vi "PC Hard.vi"(11 "DataIn":T1) -> (3 "DataOut":T1)   [LabVIEW 2017]
doc: "SubVI criada para realizar o movimento do BOT em caso de partida Player 1 x PC no nível difícil"
uses:
  controls/TabuleiroCoordenadas.ctl
  controls/GameOption.ctl
  controls/Tabuleiro.ctl
  controls/DataIn.ctl
  controls/Table.ctl
  MatchDataClasses/MatchData/MatchData.lvclass
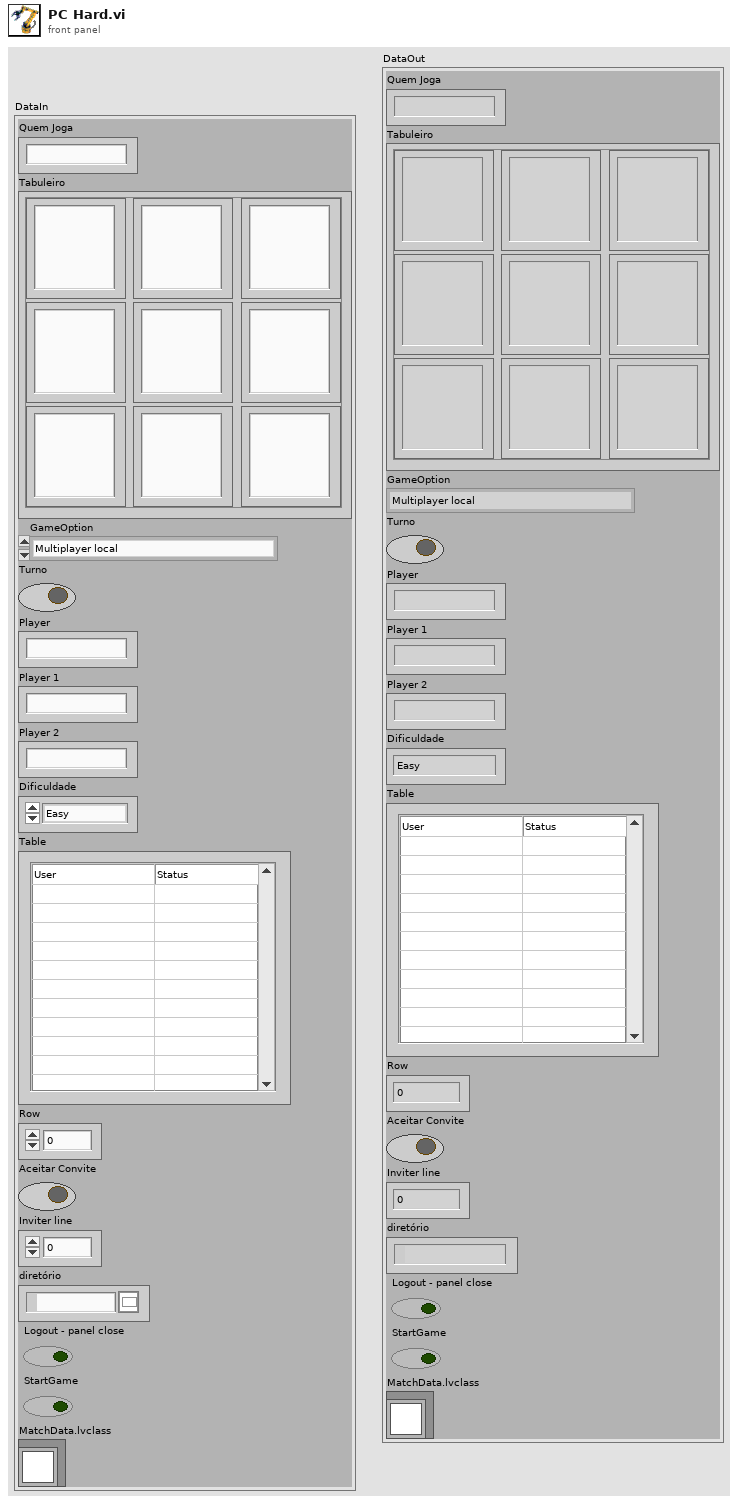
[diagram p1: front panel]
types:
  T1 = typedef "DataIn.ctl" = cluster{"Quem Joga":string, "Tabuleiro":T2, "GameOption":T3, "Turno":bool, "Player":string, "Player 1":string, "Player 2":string, "Dificuldade":enum16{"Easy", "Medium", "Hard"}, "Table":T4, "Row":u32, "Aceitar Convite":bool, "Inviter line":u32, "diretório":path, "Logout - panel close":bool, "StartGame":bool, "MatchData.lvclass":refnum<class "MatchData.lvclass">}
  T2 = typedef "Tabuleiro.ctl" = cluster{"(0,0)":string, "(1,0)":string, "(0,1)":string, "(1,1)":string, "(2,0)":string, "(1,2)":string, "(2,2)":string, "(0,2)":string, "(2,1) ":string}
  T3 = typedef "GameOption.ctl" = enum16{"Multiplayer local", "Multiplayer remoto", "Single Player", "Wait for Event", "Initialize", "Stop"}
  T4 = typedef "Table.ctl" = string[][]
  T5 = typedef "TabuleiroCoordenadas.ctl" = enum16{"0,0", "0,1", "0,2", "1,0", "1,1", "1,2", "2,0", "2,1", "2,2"}
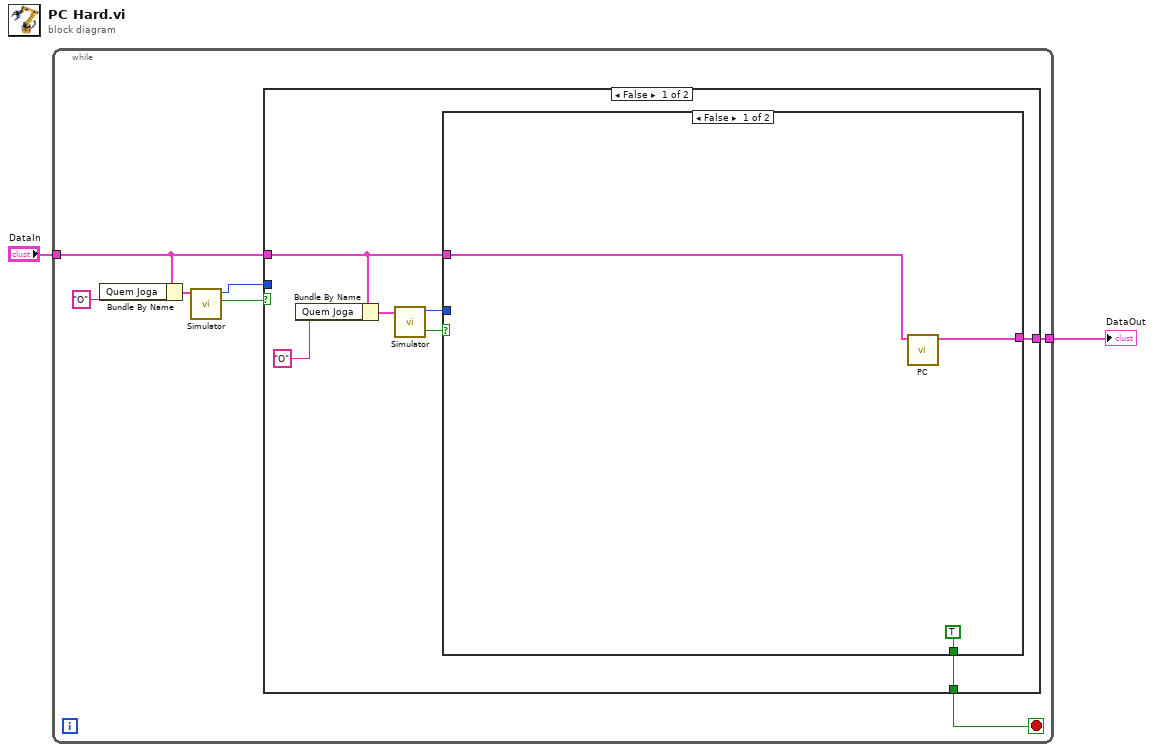
[diagram p0: block diagram]
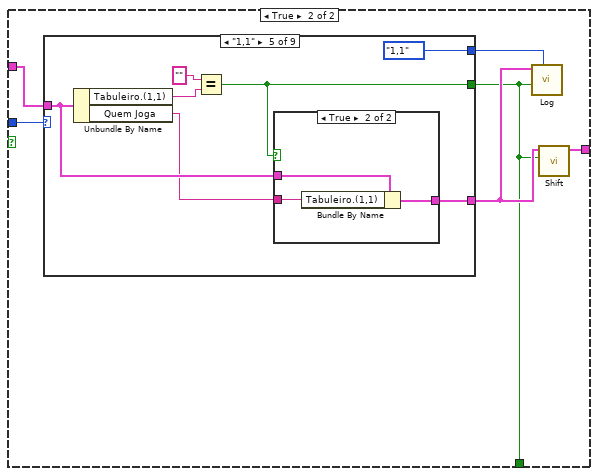
[diagram p2: hidden frame]
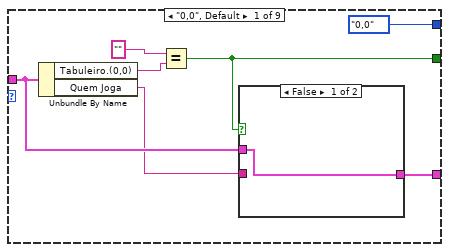
[diagram p3: hidden frame]
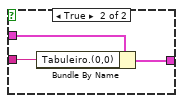
[diagram p4: hidden frame]
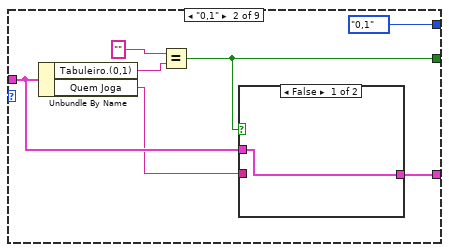
[diagram p5: hidden frame]
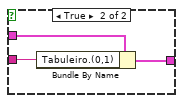
[diagram p6: hidden frame]
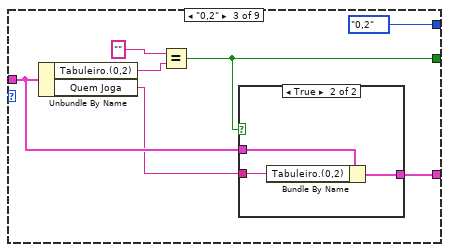
[diagram p7: hidden frame]
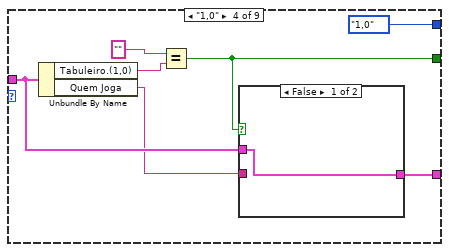
[diagram p9: hidden frame]
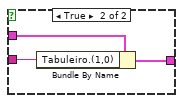
[diagram p10: hidden frame]
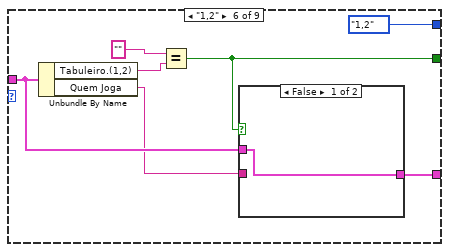
[diagram p12: hidden frame]
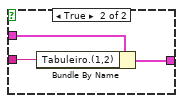
[diagram p13: hidden frame]
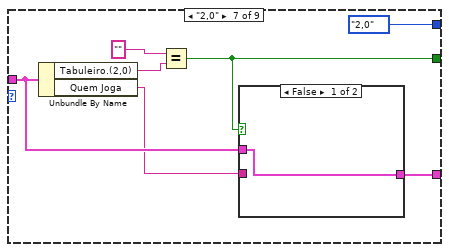
[diagram p14: hidden frame]
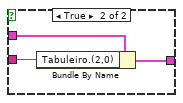
[diagram p15: hidden frame]
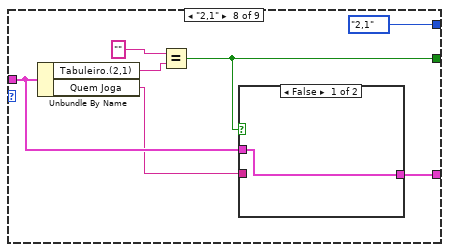
[diagram p16: hidden frame]
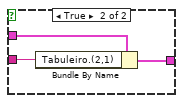
[diagram p17: hidden frame]
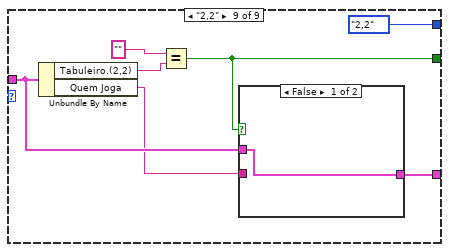
[diagram p18: hidden frame]
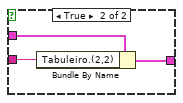
[diagram p19: hidden frame]
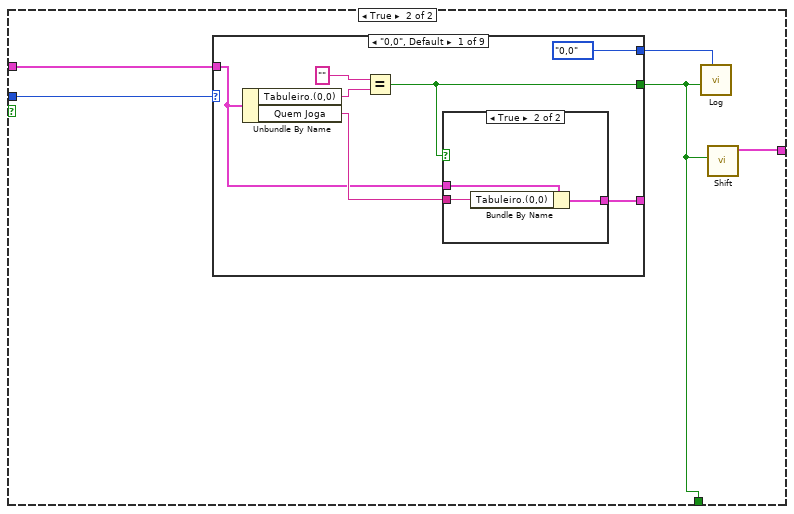
[diagram p20: hidden frame]
diagram:
  n1 = while {
    tunnel: [w9] -> w1
    tunnel: "DataIn" -> [w5]
    stop <- w4 stop-if-true
    n2 = Bundle By Name(cluster=w5, "Quem Joga"="O") -> (w6:T1)
    n3 = call "Simulator.vi"("DataIn"=w6) -> ("true = ganhou"=w8:bool, "Enum"=w3:T5)  [unwired: 9 in]
    n4 = case shown="False" w8 {
      tunnel: [w16 w129] -> w9
      tunnel: w5 -> [w11 w126]
      tunnel: [w13 w125] -> w4
      tunnel: w3 -> [_ w127]
      frame False {
        n5 = Bundle By Name(cluster=w11, "Quem Joga"="O") -> (w12:T1)
        n6 = call "Simulator.vi"("DataIn"=w12) -> ("true = ganhou"=w14:bool, "Enum"=w15:T5)  [unwired: 9 in]
        n7 = case shown="False" w14 {
          tunnel: w15 -> [_ w25]
          tunnel: w11 -> [w18 w24]
          tunnel: [w19 w21] -> w16
          tunnel: [TRUE w20] -> w13
          frame False {
            n8 = call "PC.vi"("DataIn"=w18) -> ("DataOut"=w19:T1)  [unwired: 10 in]
          }
          frame True {
            n9 = case shown="\"1,1\"" w25 {
              tunnel: w24 -> [w29 w40 w51 w62 w73 w84 w95 w106 w117]
              tunnel: [w30 w41 w52 w63 w74 w85 w96 w107 w118] -> w20
              tunnel: [w27 w38 w49 w60 w71 w82 w93 w104 w115] -> w22
              tunnel: [TabuleiroCoordenadas."0,0" ("Enum") TabuleiroCoordenadas."0,1" ("Enum") TabuleiroCoordenadas."0,2" ("Enum") TabuleiroCoordenadas."1,0" ("Enum") TabuleiroCoordenadas."1,1" ("Enum") TabuleiroCoordenadas."1,2" ("Enum") TabuleiroCoordenadas."2,0" ("Enum") TabuleiroCoordenadas."2,1" ("Enum") TabuleiroCoordenadas."2,2" ("Enum")] -> w23
              frame "0,0", Default {
                n10 = Unbundle By Name(w29) -> ("Tabuleiro.(0,0)"=w32:string, "Quem Joga"=w28:string)
                n11 = Equal?(x="", y=w32) -> (x = y?=w30:bool)
                n12 = case shown="False" w30 {
                  tunnel: w29 -> [w33 w36]
                  tunnel: w28 -> [_ w35]
                  tunnel: [w33 w34] -> w27
                  frame False {
                  }
                  frame True {
                    n13 = Bundle By Name(cluster=w36, "Tabuleiro.(0,0)"=w35) -> (w34:T1)
                  }
                }
              }
              frame "0,1" {
                n14 = Unbundle By Name(w40) -> ("Tabuleiro.(0,1)"=w43:string, "Quem Joga"=w39:string)
                n15 = Equal?(x="", y=w43) -> (x = y?=w41:bool)
                n16 = case shown="False" w41 {
                  tunnel: w40 -> [w44 w47]
                  tunnel: w39 -> [_ w46]
                  tunnel: [w44 w45] -> w38
                  frame False {
                  }
                  frame True {
                    n17 = Bundle By Name(cluster=w47, "Tabuleiro.(0,1)"=w46) -> (w45:T1)
                  }
                }
              }
              frame "0,2" {
                n18 = Unbundle By Name(w51) -> ("Tabuleiro.(0,2)"=w54:string, "Quem Joga"=w50:string)
                n19 = Equal?(x="", y=w54) -> (x = y?=w52:bool)
                n20 = case shown="True" w52 {
                  tunnel: w51 -> [w55 w58]
                  tunnel: w50 -> [_ w57]
                  tunnel: [w55 w56] -> w49
                  frame False {
                  }
                  frame True {
                    n21 = Bundle By Name(cluster=w58, "Tabuleiro.(0,2)"=w57) -> (w56:T1)
                  }
                }
              }
              frame "1,0" {
                n22 = Unbundle By Name(w62) -> ("Tabuleiro.(1,0)"=w65:string, "Quem Joga"=w61:string)
                n23 = Equal?(x="", y=w65) -> (x = y?=w63:bool)
                n24 = case shown="False" w63 {
                  tunnel: w62 -> [w66 w69]
                  tunnel: w61 -> [_ w68]
                  tunnel: [w66 w67] -> w60
                  frame False {
                  }
                  frame True {
                    n25 = Bundle By Name(cluster=w69, "Tabuleiro.(1,0)"=w68) -> (w67:T1)
                  }
                }
              }
              frame "1,1" {
                n26 = Unbundle By Name(w73) -> ("Tabuleiro.(1,1)"=w76:string, "Quem Joga"=w72:string)
                n27 = Equal?(x="", y=w76) -> (x = y?=w74:bool)
                n28 = case shown="True" w74 {
                  tunnel: w73 -> [w77 w80]
                  tunnel: w72 -> [_ w79]
                  tunnel: [w77 w78] -> w71
                  frame False {
                  }
                  frame True {
                    n29 = Bundle By Name(cluster=w80, "Tabuleiro.(1,1)"=w79) -> (w78:T1)
                  }
                }
              }
              frame "1,2" {
                n30 = Unbundle By Name(w84) -> ("Tabuleiro.(1,2)"=w87:string, "Quem Joga"=w83:string)
                n31 = Equal?(x="", y=w87) -> (x = y?=w85:bool)
                n32 = case shown="False" w85 {
                  tunnel: w84 -> [w88 w91]
                  tunnel: w83 -> [_ w90]
                  tunnel: [w88 w89] -> w82
                  frame False {
                  }
                  frame True {
                    n33 = Bundle By Name(cluster=w91, "Tabuleiro.(1,2)"=w90) -> (w89:T1)
                  }
                }
              }
              frame "2,0" {
                n34 = Unbundle By Name(w95) -> ("Tabuleiro.(2,0)"=w98:string, "Quem Joga"=w94:string)
                n35 = Equal?(x="", y=w98) -> (x = y?=w96:bool)
                n36 = case shown="False" w96 {
                  tunnel: w95 -> [w99 w102]
                  tunnel: w94 -> [_ w101]
                  tunnel: [w99 w100] -> w93
                  frame False {
                  }
                  frame True {
                    n37 = Bundle By Name(cluster=w102, "Tabuleiro.(2,0)"=w101) -> (w100:T1)
                  }
                }
              }
              frame "2,1" {
                n38 = Unbundle By Name(w106) -> ("Tabuleiro.(2,1)"=w109:string, "Quem Joga"=w105:string)
                n39 = Equal?(x="", y=w109) -> (x = y?=w107:bool)
                n40 = case shown="False" w107 {
                  tunnel: w106 -> [w110 w113]
                  tunnel: w105 -> [_ w112]
                  tunnel: [w110 w111] -> w104
                  frame False {
                  }
                  frame True {
                    n41 = Bundle By Name(cluster=w113, "Tabuleiro.(2,1)"=w112) -> (w111:T1)
                  }
                }
              }
              frame "2,2" {
                n42 = Unbundle By Name(w117) -> ("Tabuleiro.(2,2)"=w120:string, "Quem Joga"=w116:string)
                n43 = Equal?(x="", y=w120) -> (x = y?=w118:bool)
                n44 = case shown="False" w118 {
                  tunnel: w117 -> [w121 w124]
                  tunnel: w116 -> [_ w123]
                  tunnel: [w121 w122] -> w115
                  frame False {
                  }
                  frame True {
                    n45 = Bundle By Name(cluster=w124, "Tabuleiro.(2,2)"=w123) -> (w122:T1)
                  }
                }
              }
            }
            n46 = call "Log.vi"("Enum Coordenadas"=w23, "Confirmação"=w20, "DataIn"=w22) -> ()  [unwired: 7 in, 2 out]
            n47 = call "Shift.vi"("Confirmação"=w20, "DataIn"=w22) -> ("DataOut"=w21:T1)  [unwired: 7 in, 2 out]
          }
        }
      }
      frame True {
        n48 = case shown="\"0,0\", Default" w127 {
          tunnel: [w135 w146 w157 w168 w179 w190 w201 w212 w223] -> w125
          tunnel: [w133 w144 w155 w166 w177 w188 w199 w210 w221] -> _
          tunnel: [TabuleiroCoordenadas."0,0" ("Enum") TabuleiroCoordenadas."0,1" ("Enum") TabuleiroCoordenadas."0,2" ("Enum") TabuleiroCoordenadas."1,0" ("Enum") TabuleiroCoordenadas."1,1" ("Enum") TabuleiroCoordenadas."1,2" ("Enum") TabuleiroCoordenadas."2,0" ("Enum") TabuleiroCoordenadas."2,1" ("Enum") TabuleiroCoordenadas."2,2" ("Enum")] -> w128
          tunnel: w126 -> [w131 w141 w152 w163 w174 w185 w196 w207 w218]
          frame "0,0", Default {
            n49 = Unbundle By Name(w131) -> ("Tabuleiro.(0,0)"=w130:string, "Quem Joga"=w134:string)
            n50 = Equal?(x="", y=w130) -> (x = y?=w135:bool)
            n51 = case shown="True" w135 {
              tunnel: w134 -> [_ w140]
              tunnel: [w137 w139] -> w133
              tunnel: w131 -> [w137 w138]
              frame False {
              }
              frame True {
                n52 = Bundle By Name(cluster=w138, "Tabuleiro.(0,0)"=w140) -> (w139:T1)
              }
            }
          }
          frame "0,1" {
            n53 = Unbundle By Name(w141) -> ("Tabuleiro.(0,1)"=w142:string, "Quem Joga"=w145:string)
            n54 = Equal?(x="", y=w142) -> (x = y?=w146:bool)
            n55 = case shown="True" w146 {
              tunnel: w145 -> [_ w151]
              tunnel: [w148 w150] -> w144
              tunnel: w141 -> [w148 w149]
              frame False {
              }
              frame True {
                n56 = Bundle By Name(cluster=w149, "Tabuleiro.(0,1)"=w151) -> (w150:T1)
              }
            }
          }
          frame "0,2" {
            n57 = Unbundle By Name(w152) -> ("Tabuleiro.(0,2)"=w153:string, "Quem Joga"=w156:string)
            n58 = Equal?(x="", y=w153) -> (x = y?=w157:bool)
            n59 = case shown="False" w157 {
              tunnel: w156 -> [_ w162]
              tunnel: [w159 w161] -> w155
              tunnel: w152 -> [w159 w160]
              frame False {
              }
              frame True {
                n60 = Bundle By Name(cluster=w160, "Tabuleiro.(0,2)"=w162) -> (w161:T1)
              }
            }
          }
          frame "1,0" {
            n61 = Unbundle By Name(w163) -> ("Tabuleiro.(1,0)"=w164:string, "Quem Joga"=w167:string)
            n62 = Equal?(x="", y=w164) -> (x = y?=w168:bool)
            n63 = case shown="True" w168 {
              tunnel: w167 -> [_ w173]
              tunnel: [w170 w172] -> w166
              tunnel: w163 -> [w170 w171]
              frame False {
              }
              frame True {
                n64 = Bundle By Name(cluster=w171, "Tabuleiro.(1,0)"=w173) -> (w172:T1)
              }
            }
          }
          frame "1,1" {
            n65 = Unbundle By Name(w174) -> ("Tabuleiro.(1,1)"=w175:string, "Quem Joga"=w178:string)
            n66 = Equal?(x="", y=w175) -> (x = y?=w179:bool)
            n67 = case shown="True" w179 {
              tunnel: w178 -> [_ w184]
              tunnel: [w181 w183] -> w177
              tunnel: w174 -> [w181 w182]
              frame False {
              }
              frame True {
                n68 = Bundle By Name(cluster=w182, "Tabuleiro.(1,1)"=w184) -> (w183:T1)
              }
            }
          }
          frame "1,2" {
            n69 = Unbundle By Name(w185) -> ("Tabuleiro.(1,2)"=w186:string, "Quem Joga"=w189:string)
            n70 = Equal?(x="", y=w186) -> (x = y?=w190:bool)
            n71 = case shown="True" w190 {
              tunnel: w189 -> [_ w195]
              tunnel: [w192 w194] -> w188
              tunnel: w185 -> [w192 w193]
              frame False {
              }
              frame True {
                n72 = Bundle By Name(cluster=w193, "Tabuleiro.(1,2)"=w195) -> (w194:T1)
              }
            }
          }
          frame "2,0" {
            n73 = Unbundle By Name(w196) -> ("Tabuleiro.(2,0)"=w197:string, "Quem Joga"=w200:string)
            n74 = Equal?(x="", y=w197) -> (x = y?=w201:bool)
            n75 = case shown="True" w201 {
              tunnel: w200 -> [_ w206]
              tunnel: [w203 w205] -> w199
              tunnel: w196 -> [w203 w204]
              frame False {
              }
              frame True {
                n76 = Bundle By Name(cluster=w204, "Tabuleiro.(2,0)"=w206) -> (w205:T1)
              }
            }
          }
          frame "2,1" {
            n77 = Unbundle By Name(w207) -> ("Tabuleiro.(2,1)"=w208:string, "Quem Joga"=w211:string)
            n78 = Equal?(x="", y=w208) -> (x = y?=w212:bool)
            n79 = case shown="True" w212 {
              tunnel: w211 -> [_ w217]
              tunnel: [w214 w216] -> w210
              tunnel: w207 -> [w214 w215]
              frame False {
              }
              frame True {
                n80 = Bundle By Name(cluster=w215, "Tabuleiro.(2,1)"=w217) -> (w216:T1)
              }
            }
          }
          frame "2,2" {
            n81 = Unbundle By Name(w218) -> ("Tabuleiro.(2,2)"=w219:string, "Quem Joga"=w222:string)
            n82 = Equal?(x="", y=w219) -> (x = y?=w223:bool)
            n83 = case shown="True" w223 {
              tunnel: w222 -> [_ w228]
              tunnel: [w225 w227] -> w221
              tunnel: w218 -> [w225 w226]
              frame False {
              }
              frame True {
                n84 = Bundle By Name(cluster=w226, "Tabuleiro.(2,2)"=w228) -> (w227:T1)
              }
            }
          }
        }
        n85 = call "Log.vi"("Enum Coordenadas"=w128, "Confirmação"=w125) -> ()  [unwired: 8 in, 2 out]
        n86 = call "Shift.vi"("Confirmação"=w125) -> ("DataOut"=w129:T1)  [unwired: 8 in, 2 out]
      }
    }
  }
  "DataOut" <- w1
